vi "tdms test.vi"() -> ()   [LabVIEW 2013, in "tdms logger tests.lvlib"]
uses:
  tdms logger tests.lvlib
  configuration/TDMS datalogger configuration.lvclass
  execution/TDMS datalogger runtime.lvclass
  <vilib>/NI/Tag Bus Module Framework/channel/TBM channel.lvclass
  <vilib>/NI/Tag Bus Module Framework/channel/channel classification.ctl
  <vilib>/NI/Tag Bus/tag/Data Type.ctl
  <vilib>/NI/Tag Bus/tag/tag descriptor.lvclass
  <vilib>/NI/Tag Bus/table/data table.lvlib
  <vilib>/platform/TimedLoop/XDataNode/XDataNode.xnode
  <vilib>/Platform/TimedLoop/XDataNode/nitl_modes.ctl
  <vilib>/Platform/TimedLoop/XDataNode/XDNodeRunTimeDep.lvlib
  <vilib>/Platform/TimedLoop/XDataNode/wakeup.ctl
  <vilib>/Platform/TimedLoop/XDataNode/timing_clust.ctl
  <vilib>/NI/Tag Bus/table/data polymorphs/write one/write Boolean.vi
  <vilib>/Utility/RT CPU pool selections.ctl
  <vilib>/NI/Configuration Framework/serializable configuration/NISE_CEF_serializable configuration.lvclass
panel:
  out "max":dbl
  out "min":dbl
  in  "enable state":bool=TRUE
  out "found?":bool
  in  "stop":bool
  out "error out":errorcluster
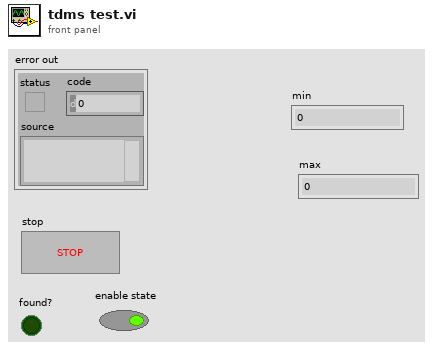
[diagram p1: front panel]
types:
  T1 = typedef "tag bus.lvlib/tag descriptor.lvclass/Data Type.ctl" = enum16{"Double", "Single", "I64", "I32", "I16", "I8", "U64", "U32", "U16", "U8", "Boolean", "String", "Array of Double", "Array of Single", "Array of I64", "Array of I32", "Array of I16", "Array of I8", "Array of U64", "Array of U32", "Array of U16", "Array of U8", "Array of Boolean", "Array of String"}
  T2 = typedef "TBM channel.lvclass/channel classification.ctl" = enum16{"input data", "output data", "processing parameter", "processing result"}
  T3 = typedef "NI_Real-Time Target Support.lvlib/RT CPU pool selections.ctl" = enum16{"System & Timed Structures", "System", "Timed Structures", "Reserved"}
  T4 = typedef "TBM channel.lvclass/data tables.ctl" = cluster{"input data":T5, "processing parameter":T5, "processing result":T5, "output data":T5}
  T5 = typedef "tag bus.lvlib/dictionary table pair.ctl" = cluster{"data dictionary":refnum<class "data dictionary.lvclass">, "data table":T6}
  T6 = typedef "tag bus.lvlib/data table.lvlib/data table.ctl" = cluster{"Double":dbl[], "Single":sgl[], "I64":i64[], "I32":i32[], "I16":i16[], "I8":i8[], "U64":u64[], "U32":u32[], "U16":u16[], "U8":u8[], "Boolean":bool[], "String":string[], "Array of Double":cluster{"DBL Array":dbl[]}[], "Array of Single":cluster{"SGL Array":sgl[]}[], "Array of I64":cluster{"I64 Array":i64[]}[], "Array of I32":cluster{"I32 Array":i32[]}[], "Array of I16":cluster{"I16 Array":i16[]}[], "Array of I8":cluster{"I8 Array":i8[]}[], "Array of U64":cluster{"U64 Array":u64[]}[], "Array of U32":cluster{"U32 Array":u32[]}[], "Array of U16":cluster{"U16 Array":u16[]}[], "Array of U8":cluster{"U8 Array":u8[]}[], "Array of Boolean":cluster{"Boolean Array":bool[]}[], "Array of String":cluster{"String Array":string[]}[]}
  T7 = typedef "XDNodeRunTimeDep.lvlib/timing_clust.ctl" = cluster{"Expected End [f-1]":u64, "Actual End [f-1]":u64, "Finished Late? [f-1]":bool, "Expected End [i-1]":u64, "Actual End [i-1]":u64, "Finished Late? [i-1]":bool, "Expected Start [i]":u64, "Actual Start [i]":u64, "Expected Start [f]":u64, "Actual Start [f]":u64, "Source Name":string, "Structure Name":string, "Period":i64, "Deadline":i64, "Offset":i64, "Start":i64, "Priority":i32, "Timeout":i32, "Mode":T8, "Wakeup Reason":T9, "Error":errorcluster, "Source Type":string, "Secondary Source Type":string, "Global End Time":u64, "Global Start Time":u64, "Frame Duration":u64, "Iteration Duration":u64, "Assigned CPU":i32, "I/O Scan Engine Mode":u32}
  T8 = typedef "XDNodeRunTimeDep.lvlib/nitl_modes.ctl" = enum32{"No Change", "Process missed periods, maintain original phase", "Discard missed periods, maintain original phase", "Process missed periods, ignore original phase", "Discard missed periods, ignore original phase"}
  T9 = typedef "XDNodeRunTimeDep.lvlib/wakeup.ctl" = enum32{"Normal", "Aborted", "Asynchronous wakeup", "Timing source error", "Timed loop error", "Timeout"}
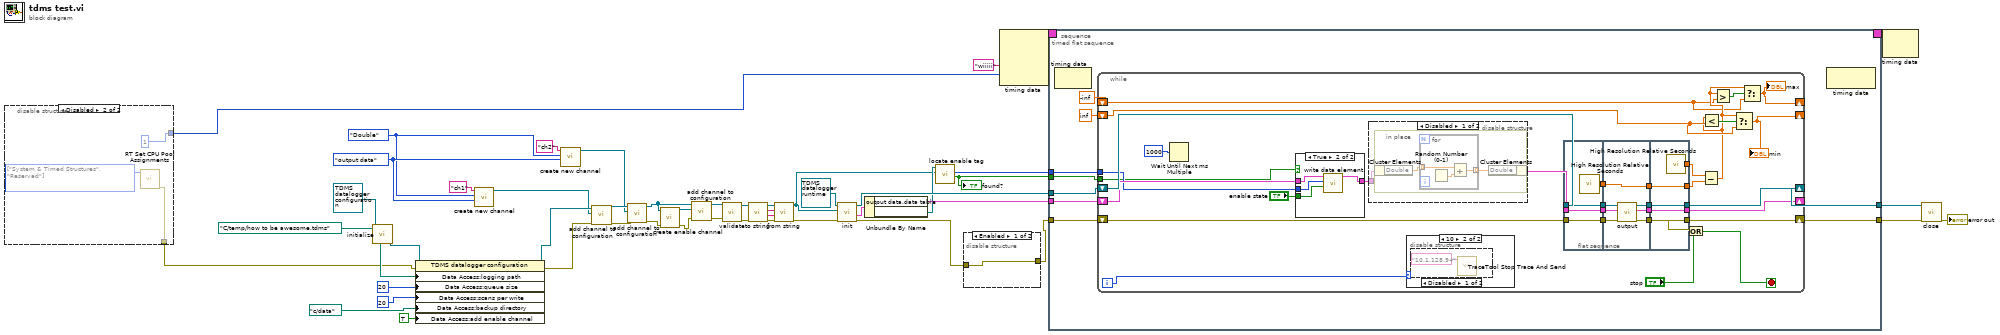
[diagram p0: block diagram]
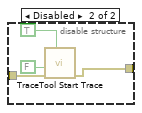
[diagram p2: hidden frame]
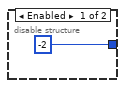
[diagram p3: hidden frame]
diagram:
  w31 = Data_Type."Double" ("data type")
  w32 = channel_classification."output data" ("channel classification")
  n1 = disable-structure shown="Disabled" {
    disable-tunnel: [_ w51] -> w19
    disable-tunnel: [-2 ("Processor") 1 ("Processor")] -> w18
    frame Enabled {
    }
    frame Disabled {
      w52 = T3[] [enum."System & Timed Structures", enum."Reserved"] items=["System & Timed Structures", "System", "Timed Structures", "Reserved"] ("CPU pools")
      n2 = call <vilib>:"RT Set CPU Pool Assignments.vi"("CPU pools"=w52) -> ("error out"=w51:errorcluster)  [unwired: 7 in, 3 out]
    }
  }
  n3 = call <vilib>:"initialize.vi"("configuration in"=refnum<class "TDMS datalogger configuration.lvclass"> refnum ("TDMS datalogger configuration")) -> ("configuration out"=w1:refnum<class "TDMS datalogger configuration.lvclass">)  [unwired: 8 in, 2 out]
  n4 = property class="TDMS datalogger configuration"(reference=w1, error in=w19, "Data Access:logging path"=path "C:/temp/how to be awesome.tdms" ("output file path"), "Data Access:queue size"=20 ("queue size"), "Data Access:scans per write"=20 ("scans per write"), "Data Access:backup directory"=path "c:/data" ("output file path"), "Data Access:add enable channel"=TRUE ("add enable channel")) -> (reference out=w11:refnum<class "TDMS datalogger configuration.lvclass">, error out=w10:errorcluster)
  n5 = call <vilib>:"create new channel.vi"("channel classification"=w32, "data type"=w31, "channel name"="ch1") -> ("channel"=w9:refnum<class "TBM channel.lvclass">)  [unwired: 8 in]
  n6 = call <vilib>:"create new channel.vi"("channel classification"=w32, "data type"=w31, "channel name"="ch2") -> ("channel"=w7:refnum<class "TBM channel.lvclass">)  [unwired: 8 in]
  n7 = call "add channel to configuration.vi"("error in"=w10, "TBM channel in"=w9, "TDMS datalogger configuration in"=w11) -> ("error out"=w8:errorcluster, "TDMS datalogger configuration out"=w12:refnum<class "TDMS datalogger configuration.lvclass">)  [unwired: 7 in]
  n8 = call "add channel to configuration.vi"("error in"=w8, "TBM channel in"=w7, "TDMS datalogger configuration in"=w12) -> ("error out"=w4:errorcluster, "TDMS datalogger configuration out"=w3:refnum<class "TDMS datalogger configuration.lvclass">)  [unwired: 7 in]
  n9 = call "create enable channel.vi"("error in"=w4, "TDMS datalogger configuration"=w3) -> ("error out"=w5:errorcluster, "enable channel"=w6:refnum<class "TBM channel.lvclass">)  [unwired: 7 in, 1 out]
  n10 = call "add channel to configuration.vi"("error in"=w5, "TBM channel in"=w6, "TDMS datalogger configuration in"=w3) -> ("error out"=w14:errorcluster, "TDMS datalogger configuration out"=w13:refnum<class "TDMS datalogger configuration.lvclass">)  [unwired: 7 in]
  n11 = call-dynamic "validate.vi"("error in"=w14, "TDMS datalogger configuration in"=w13) -> ("error out"=w48:errorcluster, "TDMS datalogger configuration out"=w47:refnum<class "TDMS datalogger configuration.lvclass">)  [unwired: 8 in]
  n12 = call-dynamic "to string.vi"("error in"=w48, "TDMS datalogger configuration in"=w47) -> ("error out"=w45:errorcluster, "data"=w44:string, "version"=w43:string, "TDMS datalogger configuration out"=w46:refnum<class "TDMS datalogger configuration.lvclass">)  [unwired: 6 in]
  n13 = call-dynamic "from string.vi"("error in"=w45, "data"=w44, "version"=w43, "TDMS datalogger configuration in"=w46) -> ("error out"=w42:errorcluster, "TDMS datalogger configuration out"=w2:refnum<class "TDMS datalogger configuration.lvclass">)  [unwired: 6 in]
  n14 = call-dynamic "init.vi"("error in"=w42, "TBM module configuration in"=w2, "TDMS datalogger runtime in"=refnum<class "TDMS datalogger runtime.lvclass"> refnum ("TDMS datalogger runtime")) -> ("error out"=w17:errorcluster, "data allocations"=w34:T4, "TDMS datalogger runtime out"=w41:refnum<class "TDMS datalogger runtime.lvclass">)  [unwired: 5 in, 1 out]
  n15 = Unbundle By Name(w34) -> ("output data.data table"=w40:T6, "output data.data dictionary"=w24:refnum<class "data dictionary.lvclass">)
  n16 = call "locate enable tag.vi"("TDMS datalogger configuration"=w2, "data dictionary in"=w24) -> ("found?"=w22:bool, "index"=w23:i32)  [unwired: 7 in, 1 out]
  "found?" <- w22
  n17 = disable-structure shown="Enabled" {
    disable-tunnel: [w53 w56] -> w16
    disable-tunnel: w17 -> [w53 w57]
    frame Enabled {
    }
    frame Disabled {
      n18 = call <vilib>:"TraceTool Start Trace.vi"("Detailed Tracing? (F)"=TRUE, "error in (no error)"=w57, "VI Tracing? (T)"=FALSE) -> ("error out"=w56:errorcluster)  [unwired: 7 in, 1 out]
    }
  }
  n19 = node-c288("wiiiii" ("Structure Name"), w18) -> (w21:T7)  [unwired: 2 in]
  n20 = timed-sequence {
    timing: w21 -> [_]
    timing-out: [_] -> w20
    tunnel: w41 -> [w64]
    tunnel: w16 -> [w63]
    tunnel: w40 -> [w62]
    tunnel: [w61] -> w39
    tunnel: [w60] -> w38
    tunnel: w23 -> [w59]
    tunnel: w22 -> [w58]
    n21 = timed-flat-sequence {
      tunnel: w64 -> [w73]
      tunnel: w63 -> [w72]
      tunnel: w62 -> [w71]
      tunnel: [w70] -> w61
      tunnel: [w69] -> w60
      tunnel: w59 -> [w68]
      tunnel: w58 -> [w67]
      n22 = node-c288() -> ()  [unwired: 1 in, 1 out]
      n23 = while {
        shift-right: [w93] -> w69
        shift-left: w72 -> [w104]
        shift-right: [w103] -> w70
        shift-left: w73 -> [w105]
        shift-right: [w101] -> _
        shift-left: w71 -> [w98]
        tunnel: w68 -> [w96]
        tunnel: w67 -> [w95]
        shift-right: [w76] -> _
        shift-left: -inf -> [w78]
        shift-right: [w77] -> _
        shift-left: inf -> [w80]
        i -> [w75]
        stop <- w94 stop-if-true
        n24 = Wait Until Next ms Multiple(millisecond multiple=u32 1000) -> ()  [unwired: 1 out]
        n25 = case shown="True" w95 {
          tunnel: w98 -> [w106 w110]
          tunnel: [w106 w109] -> w97
          tunnel: w96 -> [_ w108]
          tunnel: "enable state" -> [_ w107]
          frame False {
          }
          frame True {
            n26 = call-poly <vilib>:"write data element.vi"("value"=w107, "index"=w108, "data table in"=w110) -> ("data table out"=w109:T6)  [unwired: 8 in]
          }
        }
        n27 = disable-structure shown="Disabled" {
          disable-tunnel: [w129 w135] -> w102
          disable-tunnel: w97 -> [w128 w135]
          frame Disabled {
            n28 = in-place {
              n29 = in-place-cluster #1(w128) -> ("Double"=w131:dbl[])
              n30 = for {
                tunnel: w131 -> [w134] mode=indexing
                tunnel: [w133] -> w130 mode=indexing
                n31 = Random Number (0-1)() -> (number: 0 to 1=w132:dbl)
                n32 = Add(x=w134, y=w132) -> (x+y=w133:dbl)
              }
              n33 = in-place-cluster #1("Double"=w130) -> (w129:T6)
            }
          }
          frame Enabled {
          }
        }
        n34 = case shown="10" w75 {
          frame 0, Default {
          }
          frame 10 {
            n35 = disable-structure shown="Disabled" {
              frame Disabled {
                n36 = call <vilib>:"TraceTool Stop Trace And Send.vi"("Trace Host Network Address"="10.1.128.94") -> ()  [unwired: 10 in, 1 out]
              }
              frame Enabled {
              }
            }
          }
        }
        n37 = flat-sequence {
          tunnel: w102 -> [w113]
          tunnel: w104 -> [w114]
          tunnel: w105 -> [w115]
          tunnel: [w115] -> w89
          tunnel: [w114] -> w88
          tunnel: [w113] -> w87
          tunnel: [w112] -> w85
          tunnel: [w120] -> w92
          tunnel: [w118] -> w91
          tunnel: [w117] -> w90
          tunnel: w89 -> [w122]
          tunnel: w88 -> [w121]
          tunnel: w87 -> [w119]
          tunnel: [w116] -> w86
          tunnel: w85 -> [w116]
          tunnel: [w125] -> w93
          tunnel: [w126] -> w101
          tunnel: [w127] -> w103
          tunnel: w92 -> [w127]
          tunnel: w91 -> [w126]
          tunnel: w90 -> [w125]
          tunnel: [w124] -> w84
          tunnel: w86 -> [w124]
          tunnel: [w123] -> w83
          frame #0 {
            n38 = call <vilib>:"High Resolution Relative Seconds.vi"() -> ("relative seconds"=w112:dbl)
          }
          frame #1 {
            n39 = call-dynamic "output.vi"("error in"=w121, "data table in"=w119, "TDMS datalogger runtime in"=w122) -> ("error out"=w117:errorcluster, "data table out"=w118:T6, "TDMS datalogger runtime out"=w120:refnum<class "TDMS datalogger runtime.lvclass">)  [unwired: 6 in]
          }
          frame #2 {
            n40 = call <vilib>:"High Resolution Relative Seconds.vi"() -> ("relative seconds"=w123:dbl)
          }
        }
        n41 = Or(x=w93, y="stop") -> (x .or. y?=w94:bool)
        n42 = Subtract(x=w83, y=w84) -> (x-y=w79:dbl)
        n43 = Less?(x=w79, y=w80) -> (x < y?=w81:bool)
        n44 = Greater?(x=w79, y=w78) -> (0:w82:bool)
        n45 = Select(t=w79, s=w81, f=w80) -> (s? t:f=w77:dbl)
        "min" <- w77
        n46 = Select(t=w79, s=w82, f=w78) -> (s? t:f=w76:dbl)
        "max" <- w76
      }
      n47 = node-c288() -> ()  [unwired: 1 in, 1 out]
    }
  }
  n48 = node-c288(w20) -> ()  [unwired: 1 out]
  n49 = call-dynamic "close.vi"("error in"=w38, "TDMS datalogger runtime in"=w39) -> ("error out"=→"error out":errorcluster)  [unwired: 9 in]
